vi "NewtonsPSM_Conf_FRA.vi"(6 "Offset (0)":dbl min=-200.0 max=200.0 step=0.001, 7 "Graph (Phase)":enum16{"Phase", "Delay"}(ring), 8 "error in":errorcluster, 9 "Gain/Phase Margin (Disabled)":enum16{"Disabled", "Enabled"}(ring), 10 "Ratio (CH2/CH1)":enum16{"CH2/CH1", "CH1/CH2"}(ring), 11 "VISA.name":refnum<visa-resource-name>) -> (0 "error out":errorcluster, 3 "VISA.name out":refnum<visa-resource-name>)   [LabVIEW 2025, in "NewtonsPSM1735.lvlib"]
doc: "Set the PWM special mode to the PPA2530"
uses:
  NewtonsPSM1735.lvlib
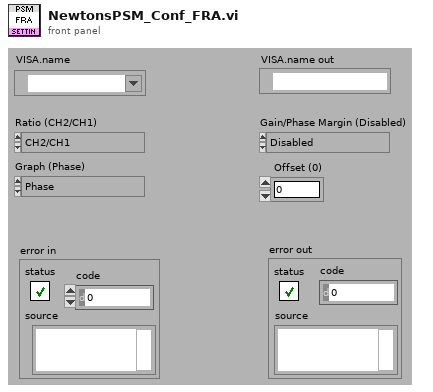
[diagram p1: front panel]
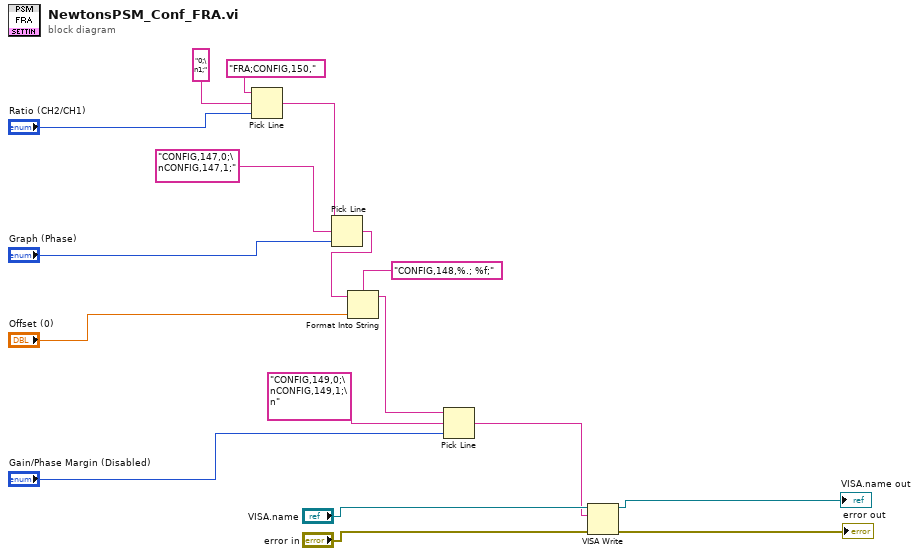
[diagram p0: block diagram]
diagram:
  n1 = Pick Line(string ("")="FRA;CONFIG,150,", multi-line string="0;\n1;", line index="Ratio (CH2/CH1)") -> (output string=w8:string)
  n2 = Pick Line(string ("")=w8, multi-line string="CONFIG,147,0;\nCONFIG,147,1;", line index="Graph (Phase)") -> (output string=w1:string)
  n3 = Format Into String(format string="CONFIG,148,%.; %f;" ("chaîne de format"), initial string=w1, "Offset (0)") -> (resulting string=w5:string)  [unwired: 1 in, 1 out]
  n4 = Pick Line(string ("")=w5, multi-line string="CONFIG,149,0;\nCONFIG,149,1;\n", line index="Gain/Phase Margin (Disabled)") -> (output string=w3:string)
  n5 = VISA Write(VISA resource name="VISA.name", write buffer=w3, error in (no error)="error in") -> (VISA resource name out=→"VISA.name out":refnum<visa-resource-name>, error out=→"error out":errorcluster)  [unwired: 1 out]
